vi "DisplacementTest.vi"() -> ()   [LabVIEW 2016]
uses:
  <vilib>/rvi/interface/nirviOpenFPGA/nirviOpenFPGA.xnode
  <vilib>/rvi/interface/nirviMethod/nirviMethod.xnode
  <vilib>/FPGAPlugInAG/Dynamic/niLvFpga_Abort_Dynamic.vi
  <vilib>/FPGAPlugInAG/Dynamic/niLvFpga_Run_Dynamic.vi
  <vilib>/rvi/interface/nirviCloseFPGA/nirviCloseFPGA.xnode
  <vilib>/FPGAPlugInAG/Dynamic/niLvFpga_Reset_Dynamic.vi
  MockDisplacementCommandFIFO/MockDisplacementlCommandFIFO.lvclass
  DisplacementDataFIFO/DisplacementDataFIFO.lvclass
  DisplacementTimestampFIFO/DisplacementTimestampFIFO.lvclass
  FPGA/RTMockDisplacement/RTMockDisplacement.lvclass
  FPGA/RTDisplacement/RTDisplacement.lvclass
  <vilib>/platform/TimedLoop/XDataNode/XDataNode.xnode
  <vilib>/Platform/TimedLoop/XDataNode/nitl_modes.ctl
  <vilib>/Platform/TimedLoop/XDataNode/XDNodeRunTimeDep.lvlib
  <vilib>/Platform/TimedLoop/XDataNode/wakeup.ctl
  <vilib>/Platform/TimedLoop/XDataNode/timing_clust.ctl
  FPGA Bitfiles/Modbus_FPGATarget_displacementTest_vId3AGE-tAs.lvbitx
  FPGA/displacementTest.vi
  <vilib>/FPGAPlugInAG/cRIO-9038/niLvFpga_Open_cRIO-9038.vi
  <vilib>/rvi/interface/common/dynamic/niFpgaDynamicAddResources.vi
  <vilib>/FPGAPlugInAG/Dynamic/niLvFpga_Close_Dynamic.vi
  D:/Code/Common_RT_FPGA/IWriteU8FIFO/IWriteU8FIFO.lvclass
  D:/Code/Common_RT_FPGA/IReadU8FIFO/IReadU8FIFO.lvclass
  D:/Code/Common_RT_FPGA/IReadU64FIFO/IReadU64FIFO.lvclass
  Scratch/RTNI9870/NI9871/NI9870.lvclass
  FPGA/RTDisplacement/DataTypes/DisplacementData.ctl
  FPGA/RTDisplacement/RTDisplacement.lvlib
panel:
  out "FPGA Error":errorcluster
  out "Read Error":errorcluster
  out "Apply Error":errorcluster
  out "DisplacementData":T1
  in  "Stop":bool
  in  "Apply":bool
  in  "Value":dbl format="%09.4f"
  in  "Sensor":u8
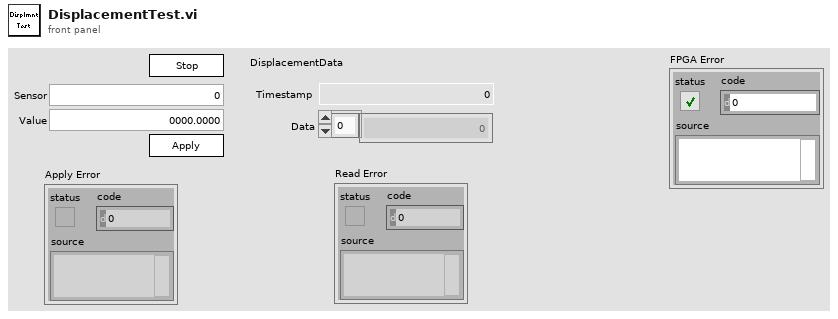
[diagram p1: front panel]
types:
  T1 = typedef "RTDisplacement.lvlib/DisplacementData.ctl" = cluster{"Timestamp":u64, "Data":dbl[]}
  T2 = typedef "XDNodeRunTimeDep.lvlib/timing_clust.ctl" = cluster{"Expected End [f-1]":u64, "Actual End [f-1]":u64, "Finished Late? [f-1]":bool, "Expected End [i-1]":u64, "Actual End [i-1]":u64, "Finished Late? [i-1]":bool, "Expected Start [i]":u64, "Actual Start [i]":u64, "Expected Start [f]":u64, "Actual Start [f]":u64, "Source Name":string, "Structure Name":string, "Period":i64, "Deadline":i64, "Offset":i64, "Start":i64, "Priority":i32, "Timeout":i32, "Mode":T3, "Wakeup Reason":T4, "Error":errorcluster, "Source Type":string, "Secondary Source Type":string, "Global End Time":u64, "Global Start Time":u64, "Frame Duration":u64, "Iteration Duration":u64, "Assigned CPU":i32, "I/O Scan Engine Mode":u32}
  T3 = typedef "XDNodeRunTimeDep.lvlib/nitl_modes.ctl" = enum32{"No Change", "Process missed periods, maintain original phase", "Discard missed periods, maintain original phase", "Process missed periods, ignore original phase", "Discard missed periods, ignore original phase"}
  T4 = typedef "XDNodeRunTimeDep.lvlib/wakeup.ctl" = enum32{"Normal", "Aborted", "Asynchronous wakeup", "Timing source error", "Timed loop error", "Timeout"}
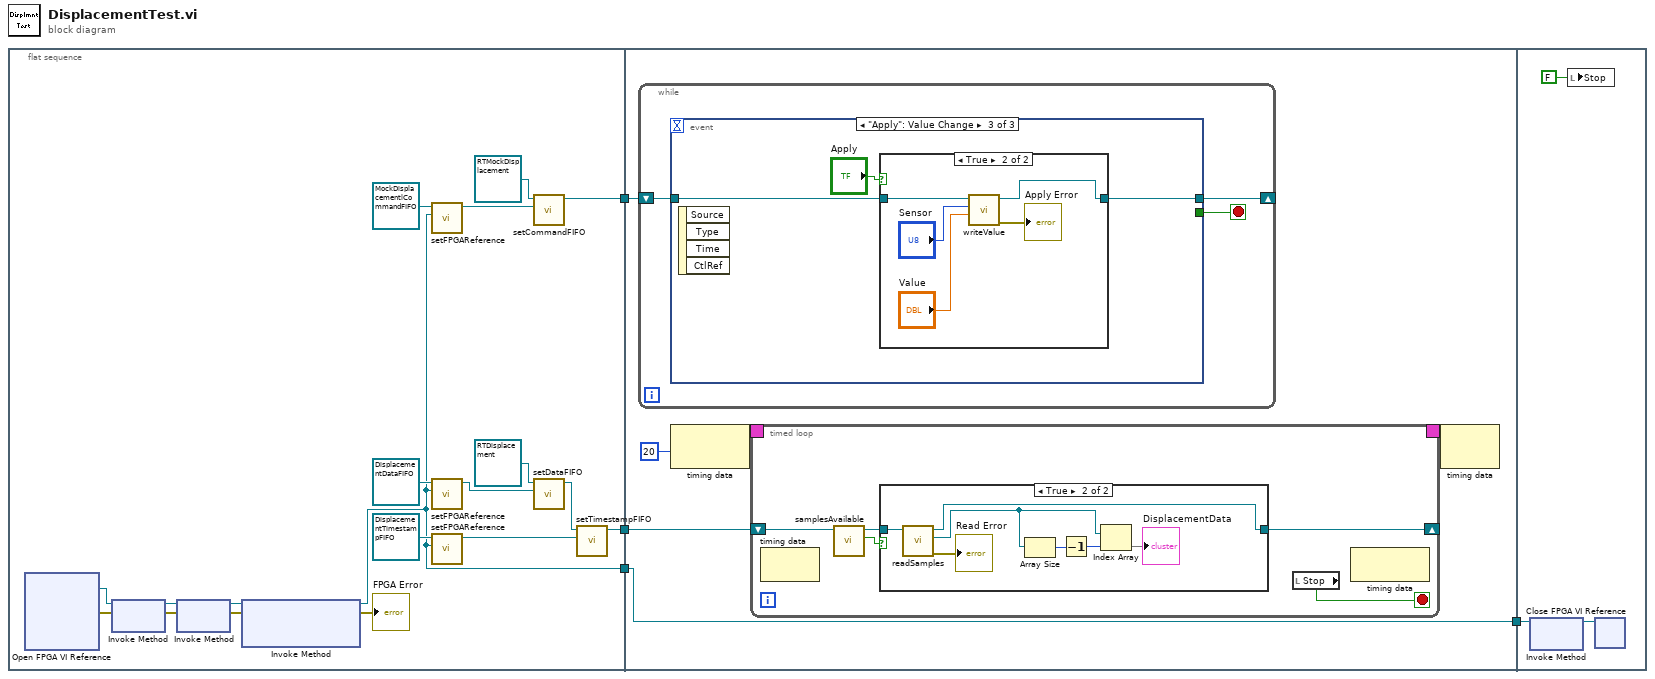
[diagram p0: block diagram]
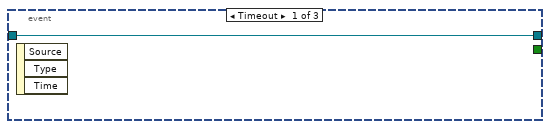
[diagram p2: hidden frame]
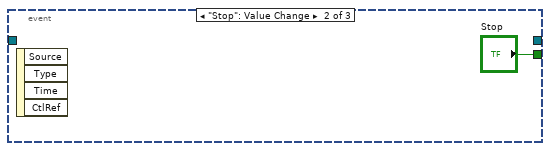
[diagram p3: hidden frame]
diagram:
  n1 = flat-sequence {
    tunnel: [w8] -> w4
    tunnel: [w7] -> w2
    tunnel: [w6] -> w1
    tunnel: w4 -> [w29]
    tunnel: [w29] -> w3
    tunnel: w2 -> [w25]
    tunnel: w1 -> [w24]
    tunnel: w3 -> [w64]
    frame #0 {
      n2 = xnode "Open FPGA VI Reference"() -> ("FPGA VI Reference Out"=w21:refnum<k20>, "error out"=w18:errorcluster)  [unwired: 2 in]
      n3 = xnode "Invoke Method"("FPGA VI Reference In"=w21, "error in"=w18) -> ("FPGA VI Reference Out"=w23:refnum<k20>, "error out"=w22:errorcluster)
      n4 = xnode "Invoke Method"("FPGA VI Reference In"=w23, "error in"=w22) -> ("FPGA VI Reference Out"=w20:refnum<k20>, "error out"=w19:errorcluster)
      n5 = xnode "Invoke Method"("FPGA VI Reference In"=w20, "error in"=w19) -> ("FPGA VI Reference Out"=w8:refnum<k20>, "error out"=→"FPGA Error":errorcluster)  [unwired: 1 in]
      n6 = call "setFPGAReference.vi"("FPGAReference"=w8, "MockDisplacementCommandFIFO in"=refnum<class "MockDisplacementlCommandFIFO.lvclass"> refnum ("MockDisplacementlCommandFIFO.lvclass")) -> ("MockDisplacementCommandFIFO out"=w13:refnum<class "MockDisplacementlCommandFIFO.lvclass">)  [unwired: 9 in]
      n7 = call "setFPGAReference.vi"("FPGAReference"=w8, "MyHealthAndStatusReadFIFO in"=refnum<class "DisplacementDataFIFO.lvclass"> refnum ("DisplacementDataFIFO.lvclass")) -> ("MyHealthAndStatusReadFIFO out"=w9:refnum<class "DisplacementDataFIFO.lvclass">)  [unwired: 9 in]
      n8 = call "setFPGAReference.vi"("FPGAReference"=w8, "MyHealthAndStatusReadFIFO in"=refnum<class "DisplacementTimestampFIFO.lvclass"> refnum ("DisplacementTimestampFIFO.lvclass")) -> ("MyHealthAndStatusReadFIFO out"=w10:refnum<class "DisplacementTimestampFIFO.lvclass">)  [unwired: 9 in]
      n9 = call "setCommandFIFO.vi"("CommandFIFO"=w13, "RTMockDisplacement in"=refnum<class "RTMockDisplacement.lvclass"> refnum ("RTMockDisplacement.lvlib:RTMockDisplacement.lvclass")) -> ("RTMockDisplacement out"=w6:refnum<class "RTMockDisplacement.lvclass">)  [unwired: 9 in]
      n10 = call "setDataFIFO.vi"("DataFIFO"=w9, "RTDisplacement in"=refnum<class "RTDisplacement.lvclass"> refnum ("RTDisplacement.lvlib:RTDisplacement.lvclass")) -> ("RTDisplacement out"=w11:refnum<class "RTDisplacement.lvclass">)  [unwired: 9 in]
      n11 = call "setTimestampFIFO.vi"("TimestampFIFO"=w10, "RTDisplacement in"=w11) -> ("RTDisplacement out"=w7:refnum<class "RTDisplacement.lvclass">)  [unwired: 9 in]
    }
    frame #1 {
      n12 = while {
        shift-right: [w31] -> _
        shift-left: w24 -> [w32]
        stop <- w30 stop-if-true
        n13 = event shown="[2] \"Apply\": Value Change" {
          selector: _ -> [_ _ _]
          dyn-events: _ -> [_ _ _]
          timeout: _ -> [_ _ _]
          tunnel: w32 -> [w33 _ w36]
          tunnel: [w33 _ w35] -> w31
          tunnel: [_ "Stop" _] -> w30
          event Timeout {
            n14 = event-data() -> ()  [unwired: 1 in, 3 out]
          }
          event "Stop": Value Change {
            n15 = event-data() -> ()  [unwired: 1 in, 4 out]
          }
          event "Apply": Value Change {
            n16 = event-data() -> ()  [unwired: 1 in, 4 out]
            n17 = case shown="True" "Apply" {
              tunnel: w36 -> [w38 w43]
              tunnel: [w38 w40] -> w35
              frame False {
              }
              frame True {
                n18 = call "writeValue.vi"("Value"="Value", "Sensor"="Sensor", "RTMockDisplacement in"=w43) -> ("error out"=→"Apply Error":errorcluster, "RTMockDisplacement out"=w40:refnum<class "RTMockDisplacement.lvclass">)  [unwired: 7 in]
              }
            }
          }
        }
      }
      n19 = node-c288(i64 20 ("Period")) -> (w28:T2)
      n20 = timed-loop {
        timing: w28 -> [_]
        timing-out: [_] -> w27
        shift-right: [w46] -> _
        shift-left: w25 -> [w47]
        stop <- w44 stop-if-true
        n21 = node-c288() -> ()  [unwired: 1 in, 1 out]
        n22 = call "samplesAvailable.vi"("RTDisplacement in"=w47) -> ("SamplesAvailable"=w45:bool, "RTDisplacement out"=w48:refnum<class "RTDisplacement.lvclass">)  [unwired: 8 in, 1 out]
        n23 = case shown="True" w45 {
          tunnel: w48 -> [w49 w52]
          tunnel: [w49 w51] -> w46
          frame False {
          }
          frame True {
            n24 = call "readSamples.vi"("RTDisplacement in"=w52) -> ("error out"=→"Read Error":errorcluster, "NI9870 out"=w54:refnum<class "NI9870.lvclass">, "RTDisplacement out"=w51:refnum<class "RTDisplacement.lvclass">)  [unwired: 7 in, 1 out]
            n25 = Array Size(array=w54) -> (size(s)=w56:i32)
            n26 = Decrement(x=w56) -> (x-1=w55:i32)
            n27 = Index Array(array=w54, index=w55) -> (element=→"DisplacementData")
          }
        }
        n28 = local read "Stop"() -> (w44:bool)
        n29 = node-c288() -> ()  [unwired: 1 in, 1 out]
      }
      n30 = node-c288(w27) -> ()  [unwired: 1 out]
    }
    frame #2 {
      n31 = xnode "Invoke Method"("FPGA VI Reference In"=w64) -> ("FPGA VI Reference Out"=w65:refnum<k20>)  [unwired: 1 in, 1 out]
      n32 = local write "Stop"(FALSE ("Stop")) -> ()
      n33 = xnode "Close FPGA VI Reference"("FPGA VI Reference In"=w65) -> ()  [unwired: 1 in, 1 out]
    }
  }
